vi "Remove Invalid Scalars.vi"(8 "error in (no error)":errorcluster, 9 "Invalid":T1[](array[typedef]) {"Data Type" format="%.0x"}, 10 "Section Name":string="Scalar Inputs", 11 "Item Ref in":T3 format="%.0x") -> (0 "error out":errorcluster, 3 "Item Ref out":T3 format="%.0x")   [LabVIEW 2018, in "FPGA Addon System Explorer.lvlib"]
uses:
  FPGA Addon System Explorer.lvlib
  <vilib>/NI Veristand/Custom Device API/Custom Device Item Ref.ctl
  Addon Shared/Types/Register Information.ctl
  Addon Shared/Types/Data Type.ctl
  <vilib>/NI Veristand/Custom Device Tools/Custom Device Utility Library/NI VeriStand - Search for Item by Name.vi
  <vilib>/NI Veristand/Custom Device Tools/Custom Device Utility Library/Custom Device Utility Library.lvlib
  <vilib>/NI Veristand/Custom Device API/Custom Device API.lvlib
  Addon Shared/FPGA Addon Shared.lvlib
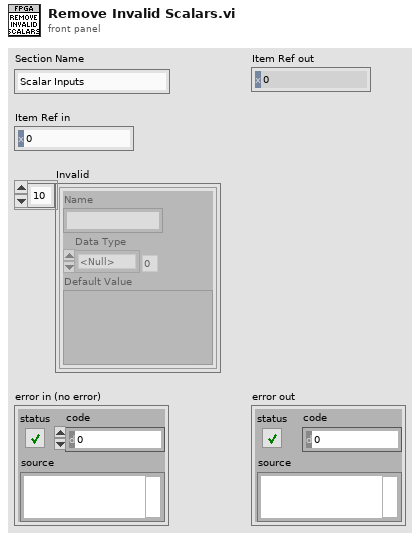
[diagram p1: front panel]
types:
  T1 = typedef "FPGA Addon Shared.lvlib/Register Information.ctl" = cluster{"Name":string, "Data Type":T2, "Default Value":variant}
  T2 = typedef "FPGA Addon Shared.lvlib/Data Type.ctl" = enum8{"<Null>", "I8", "I16", "I32", "I64", "U8", "U16", "U32", "U64", "SGL", "Boolean", "Analog PWM In Settings", "Analog PWM In", "Digital PWM In Settings", "Digital PWM In", "Digital PWM Out", "Sine Out", "FXP+/-24.5", "FXP+/-16.5", "FXP+/-32.8", "FXP+/-64.32", "FXP+/-16.7", "FXP+/-20.5", "FXP+/-27.5", "FXP+/-32.16", "FXP+16.3", "FXP+18.3", "Digital Static In", "Digital Static Out", "Digital Static In Settings", "Digital WSS Out", "Quad Encoder Settings", "Quad Encoder In", "Group"}
  T3 = typedef "Custom Device API.lvlib/Custom Device Item Ref.ctl" = u64
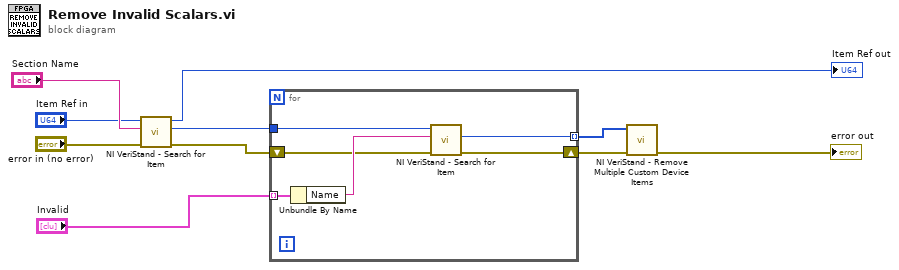
[diagram p0: block diagram]
diagram:
  n1 = call-poly <vilib>:"NI VeriStand - Search for Item.vi"("error in"="error in (no error)", "Item Name"="Section Name", "Section Ref in"="Item Ref in") -> ("error out"=w7:errorcluster, "Item Ref"=w6:T3, "Section Ref out"=→"Item Ref out":T3)  [unwired: 5 in, 1 out]
  n2 = for {
    tunnel: w6 -> [w16]
    tunnel: "Invalid" -> [w15] mode=indexing
    shift-right: [w12] -> w9
    shift-left: w7 -> [w13]
    tunnel: [w11] -> w8 mode=indexing
    n3 = Unbundle By Name(w15) -> ("Name"=w14:string)
    n4 = call-poly <vilib>:"NI VeriStand - Search for Item.vi"("error in"=w13, "Item Name"=w14, "Section Ref in"=w16) -> ("error out"=w12:errorcluster, "Item Ref"=w11:T3)  [unwired: 5 in, 2 out]
  }
  n5 = call <vilib>:"NI VeriStand - Remove Multiple Custom Device Items.vi"("error in (no error)"=w9, "Item Refs in"=w8) -> ("error out"=→"error out":errorcluster)  [unwired: 8 in, 1 out]
